vi "Simple H5Dread (Variant).vi"(4 "Data":variant, 7 "Close dataset (T)":bool=TRUE, 8 "error in (no error)":errorcluster, 10 "Dataset Path":string, 11 "HDF5 Ref":T1) -> (0 "error out":errorcluster, 1 "Data out":variant, 2 "HDF5 Dataset Ref":T1, 3 "HDF5 Ref out":T1)   [LabVIEW 2017]
doc: "Reads data from a dataset into a buffer."
uses:
  <vilib>/UPVI/lvhdf5/library.llb/HDF5 Ref.ctl
  <vilib>/UPVI/lvhdf5/common.llb/To HDF5 Ref.vi
panel:
  # "LVHDF5 Toolkit\nCopyright (c) 2005-2013 by Jason D. Sommerville\nCopyright (c) 2014 by UPVI, LLC.\n\nThis use and distribution of this file is governed by the terms found in \nLICENSE.txt distributed with this toolkit and installed at\n <user.lib>\\_lvhdf5\\LICENSE.txt"
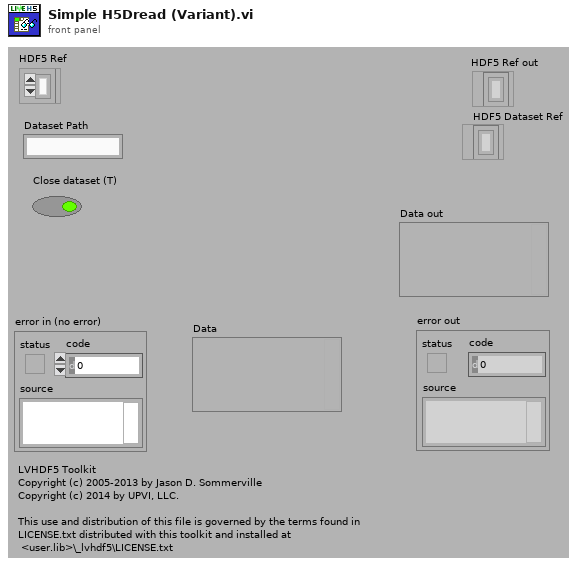
[diagram p1: front panel]
types:
  T1 = typedef "HDF5 Ref.ctl" = refnum<k1>
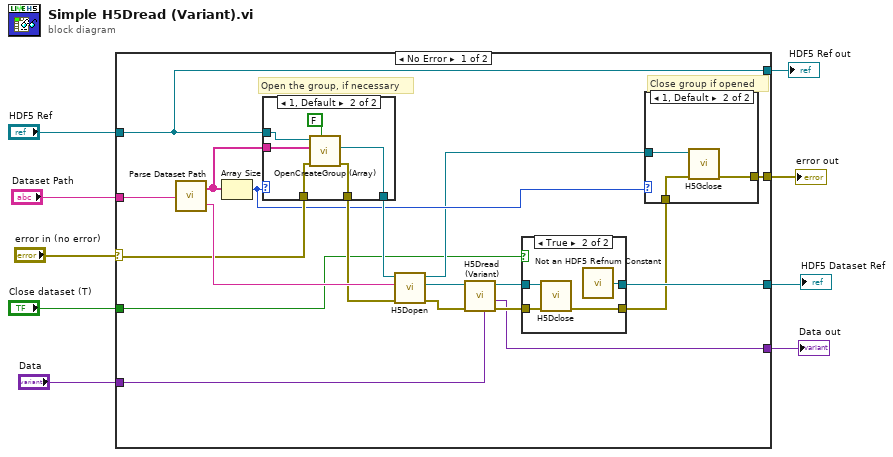
[diagram p0: block diagram]
diagram:
  n1 = case shown="No Error" "error in (no error)" {
    selector: "error in (no error)" -> [w21 w49]
    tunnel: [w16 w49] -> w8
    tunnel: "HDF5 Ref" -> [w13 w47]
    tunnel: [w14 variant ("Data")] -> w6
    tunnel: [w24 _] -> w5
    tunnel: [w13 w47] -> w4
    tunnel: "Dataset Path" -> [w12 _]
    tunnel: "Data" -> [w11 _]
    tunnel: "Close dataset (T)" -> [w10 _]
    frame No Error {
      # "Close group if opened"
      # "Open the group, if necessary"
      n2 = call <vilib>:"Parse Dataset Path.vi"("Dataset path"=w12) -> ("Groups"=w22:string[], "Dataset"=w23:string)
      n3 = Array Size(array=w22) -> (size(s)=w17:i32)
      n4 = case shown="1, Default" w17 {
        tunnel: w22 -> [_ w39]
        tunnel: w13 -> [w34 w38]
        tunnel: w21 -> [w33 w37]
        tunnel: [w33 w36] -> w20
        tunnel: [w34 w35] -> w19
        frame 0 {
        }
        frame 1, Default {
          n5 = call <vilib>:"OpenCreateGroup (Array).vi"("Create if not found (F)"=FALSE ("Create if not found (T)"), "error in (no error)"=w37, "Array of Groups"=w39, "HDF5 Ref"=w38) -> ("error out"=w36:errorcluster, "HDF5 Group Ref"=w35:T1)  [unwired: 5 in, 1 out]
        }
      }
      n6 = call <vilib>:"H5Dopen.vi"("error in (no error)"=w20, "name"=w23, "HDF5 Ref"=w19) -> ("error out"=w27:errorcluster, "HDF5 Dataset Ref"=w28:T1, "HDF5 Ref out"=w15:T1)  [unwired: 4 in]
      n7 = call <vilib>:"H5Dread (Variant).vi"("Data"=w11, "error in (no error)"=w27, "HDF5 Dataset Ref"=w28) -> ("error out"=w25:errorcluster, "Data out"=w14:variant, "HDF5 Dataset Ref out"=w26:T1)  [unwired: 6 in]
      n8 = case shown="True" w10 {
        tunnel: w26 -> [w41 w46]
        tunnel: w25 -> [w42 w45]
        tunnel: [w42 w44] -> w18
        tunnel: [w41 w43] -> w24
        frame False {
        }
        frame True {
          n9 = call <vilib>:"H5Dclose.vi"("error in (no error)"=w45, "HDF5 Dataset Ref"=w46) -> ("error out"=w44:errorcluster)  [unwired: 7 in]
          n10 = call <vilib>:"Not an HDF5 Refnum Constant.vi"() -> ("HDF5 Ref"=w43:T1)
        }
      }
      n11 = case shown="1, Default" w17 {
        tunnel: w18 -> [w29 w32]
        tunnel: [w29 w31] -> w16
        tunnel: w15 -> [_ w30]
        frame 0 {
        }
        frame 1, Default {
          n12 = call <vilib>:"H5Gclose.vi"("error in (no error)"=w32, "HDF5 Group Ref"=w30) -> ("error out"=w31:errorcluster)  [unwired: 7 in]
        }
      }
    }
    frame Error {
    }
  }
  "error out" <- w8
  "HDF5 Ref out" <- w4
  "Data out" <- w6
  "HDF5 Dataset Ref" <- w5
